vi "03Foot_CompressWave.vi"(11 "Input":dbl[](array[numeric])) -> (3 "Output":dbl[](array[numeric]))   [LabVIEW 2015]
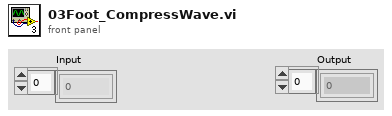
[diagram p1: front panel]
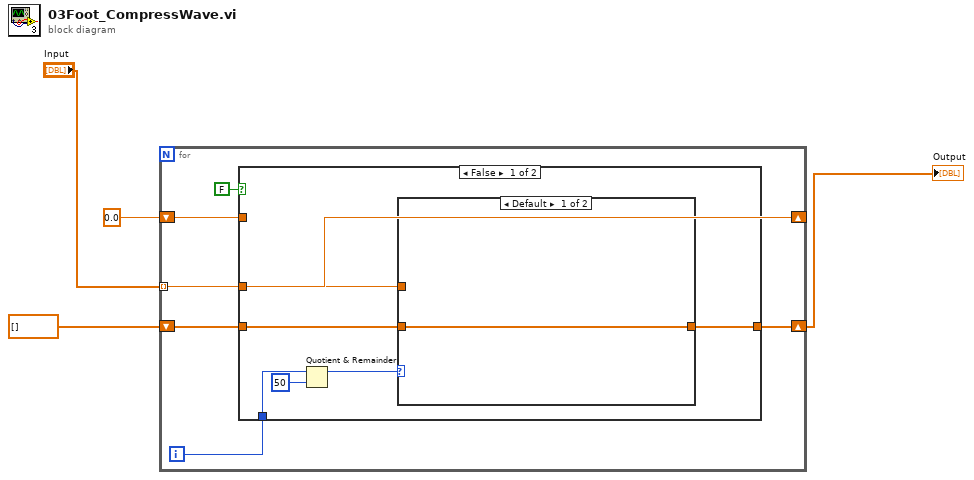
[diagram p0: block diagram]
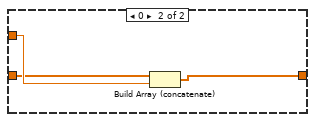
[diagram p2: hidden frame]
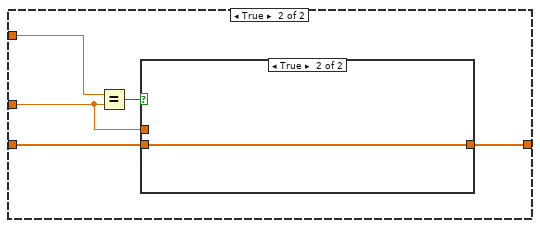
[diagram p3: hidden frame]
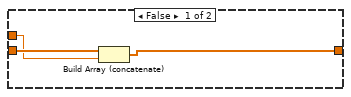
[diagram p4: hidden frame]
diagram:
  n1 = for {
    tunnel: "Input" -> [w9] mode=indexing
    shift-right: [w9] -> _
    shift-left: 0.0 -> [w10]
    shift-right: [w7] -> w1
    shift-left: dbl[] [] -> [w8]
    i -> [w5]
    n2 = case shown="False" FALSE {
      tunnel: w10 -> [_ w24]
      tunnel: w9 -> [w12 w23]
      tunnel: w8 -> [w13 w22]
      tunnel: [w14 w21] -> w7
      tunnel: w5 -> [w16 _]
      frame False {
        n3 = Quotient & Remainder(x=w16, y=50) -> (x-y*floor(x/y)=w11:i32)  [unwired: 1 out]
        n4 = case shown="Default" w11 {
          tunnel: [w17 w18] -> w14
          tunnel: w13 -> [w17 w19]
          tunnel: w12 -> [_ w20]
          frame Default {
          }
          frame 0 {
            n5 = Build Array (concatenate)(w19, w20) -> (w18:dbl[])
          }
        }
      }
      frame True {
        n6 = Equal?(x=w24, y=w23) -> (x = y?=w25:bool)
        n7 = case shown="True" w25 {
          tunnel: w23 -> [w26 _]
          tunnel: w22 -> [w28 w29]
          tunnel: [w27 w29] -> w21
          frame False {
            n8 = Build Array (concatenate)(w28, w26) -> (w27:dbl[])
          }
          frame True {
          }
        }
      }
    }
  }
  "Output" <- w1
